vi "test_Put and Get file.vi"(8 "error in (no error)":errorcluster, 11 "TestCase in":refnum<class "[Test Case] Put and Get file.lvclass">) -> (0 "error out":errorcluster, 3 "TestCase out":refnum<class "[Test Case] Put and Get file.lvclass">)   [LabVIEW 2015, in "Tests.lvlib" / "[Test Case] Put and Get file.lvclass"]
uses:
  [Test Case] Put and Get file.lvclass
  [Test Case] Put and Get file.lvclass/[Test Case] Put and Get file.ctl
  classes/File Transfer Behavior/Type.ctl
  classes/File Transfer Behavior/File Transfer Behavior.lvclass
  <vilib>/addons/_JKI Toolkits/VI Tester/TestCase.llb/TestCase.lvclass
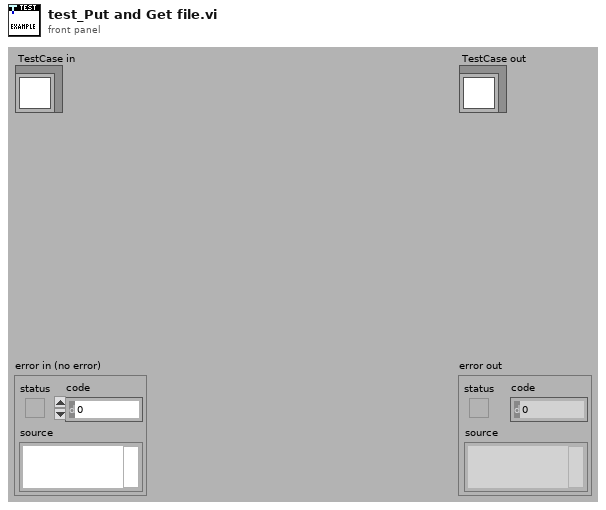
[diagram p1: front panel]
types:
  T1 = typedef "RT Management.lvlib/File Transfer Behavior.lvclass/Type.ctl" = enum16{"unknown", "file", "directory"}
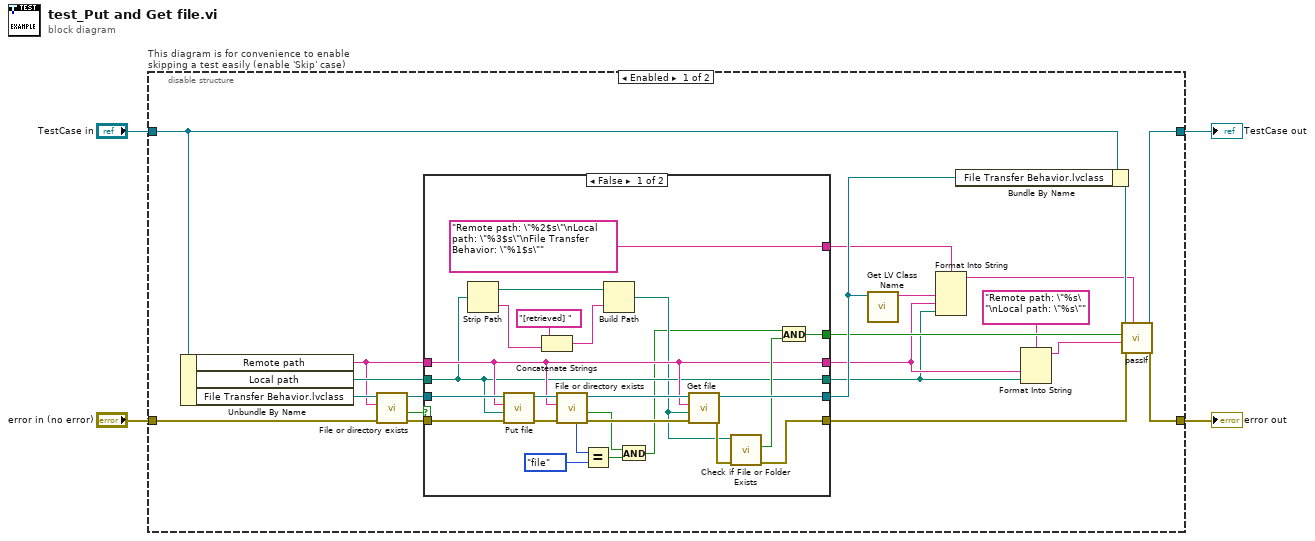
[diagram p0: block diagram]
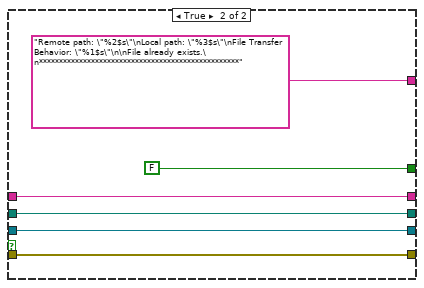
[diagram p2: hidden frame]
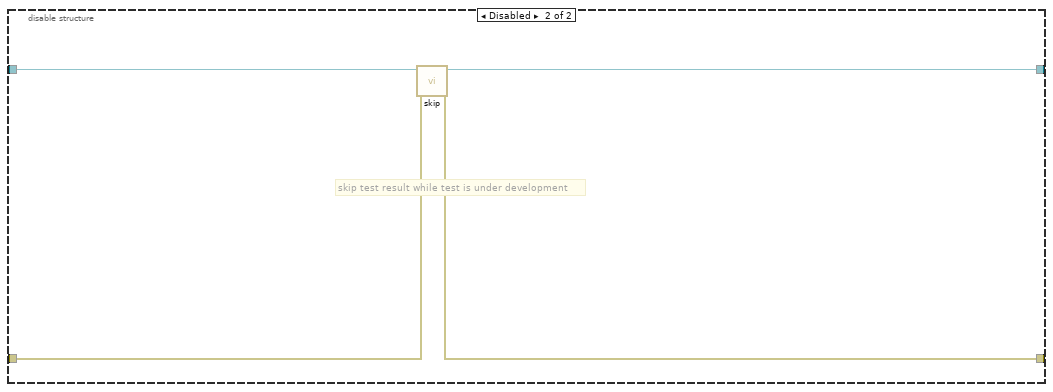
[diagram p3: hidden frame]
diagram:
  n1 = disable-structure "This diagram is for convenience to enable skipping a test easily (enable 'Skip' case)" shown="Enabled" {
    disable-tunnel: "TestCase in" -> [w12 w59]
    disable-tunnel: [w22 w57] -> w1
    disable-tunnel: [w21 w58] -> w3
    disable-tunnel: "error in (no error)" -> [w17 w56]
    frame Enabled {
      n2 = Unbundle By Name(w12) -> ("Remote path"=w15:string, "Local path"=w23:path, "File Transfer Behavior.lvclass"=w16:refnum<class "File Transfer Behavior.lvclass">)
      n3 = call-dynamic "File or directory exists.vi"("error in (no error)"=w17, "Path"=w15, "File Transfer Behavior in"=w16) -> ("error out"=w18:errorcluster, "Exists?"=w14:bool, "File Transfer Behavior out"=w24:refnum<class "File Transfer Behavior.lvclass">)  [unwired: 4 in, 2 out]
      n4 = case shown="False" w14 {
        tunnel: w24 -> [w48 w52]
        tunnel: w23 -> [w28 w53]
        tunnel: [w32 FALSE] -> w20
        tunnel: [w30 w51] -> w19
        tunnel: w18 -> [w42 w51]
        tunnel: w15 -> [w29 w54]
        tunnel: [w49 w52] -> w25
        tunnel: ["Remote path: \"%2$s\"\nLocal path: \"%3$s\"\nFile Transfer Behavior: \"%1$s\"" ("format string") "Remote path: \"%2$s\"\nLocal path: \"%3$s\"\nFile Transfer Behavior: \"%1$s\"\n\nFile already exists.\n**************************************************" ("format string")] -> w9
        tunnel: [w29 w54] -> w8
        tunnel: [w28 w53] -> w7
        frame False {
          n5 = Strip Path(path=w28) -> (stripped path=w36:path, name=w34:string)
          n6 = call-dynamic "Put file.vi"("error in (no error)"=w42, "Local path"=w28, "Remote path"=w29, "File Transfer Behavior in"=w48) -> ("error out"=w47:errorcluster, "File Transfer Behavior out"=w46:refnum<class "File Transfer Behavior.lvclass">)  [unwired: 6 in]
          n7 = Concatenate Strings("[retrieved] " ("string"), w34) -> (w35:string)
          n8 = call-dynamic "File or directory exists.vi"("error in (no error)"=w47, "Path"=w29, "File Transfer Behavior in"=w46) -> ("error out"=w40:errorcluster, "Exists?"=w38:bool, "File Transfer Behavior out"=w39:refnum<class "File Transfer Behavior.lvclass">, "Type"=w45:T1)  [unwired: 4 in, 1 out]
          n9 = Equal?(x=w45, y=Type."file" ("Type")) -> (x = y?=w43:bool)
          n10 = Build Path(base path=w36, name or relative path=w35) -> (appended path=w27:path)
          n11 = And(x=w38, y=w43) -> (x .and. y?=w26:bool)
          n12 = call-dynamic "Get file.vi"("error in (no error)"=w40, "Local path"=w27, "Remote path"=w29, "File Transfer Behavior in"=w39) -> ("error out"=w33:errorcluster, "File Transfer Behavior out"=w49:refnum<class "File Transfer Behavior.lvclass">)  [unwired: 6 in]
          n13 = call <vilib>:"Check if File or Folder Exists.vi"("error in (no error)"=w33, "path"=w27) -> ("error out"=w30:errorcluster, "file or folder exists?"=w31:bool)  [unwired: 7 in, 1 out]
          n14 = And(x=w26, y=w31) -> (x .and. y?=w32:bool)
        }
        frame True {
        }
      }
      n15 = call <vilib>:"Get LV Class Name.vi"("object"=w25) -> ("class name"=w13:string)  [unwired: 9 in, 1 out]
      n16 = Format Into String(format string=w9, w13, w8, w7) -> (resulting string=w10:string)  [unwired: 2 in, 1 out]
      n17 = Bundle By Name(cluster=w12, "File Transfer Behavior.lvclass"=w25) -> (w11:refnum<class "[Test Case] Put and Get file.lvclass">)
      n18 = Format Into String(format string="Remote path: \"%s\"\nLocal path: \"%s\"", w8, w7) -> (resulting string=w5:string)  [unwired: 2 in, 1 out]
      n19 = call-dynamic "passIf.vi"("custom report message (\"\")"=w10, "error in (no error)"=w19, "message (\"\")"=w5, "pass"=w20, "TestCase in"=w11) -> ("error out"=w21:errorcluster, "TestCase out"=w22:refnum<class "[Test Case] Put and Get file.lvclass">)  [unwired: 5 in]
    }
    frame Disabled {
      # "skip test result while test is under development"
      n20 = call <vilib>:"skip.vi"("error in (no error)"=w56, "TestCase in"=w59) -> ("error out"=w58:errorcluster, "TestCase out"=w57:refnum<class "[Test Case] Put and Get file.lvclass">)  [unwired: 8 in]
    }
  }
  "error out" <- w3
  "TestCase out" <- w1
